vi "DSF.Engine.BuilderManager.Get Builder FIFO.vi"(11 "Builder Manager in":refnum<class "DSF.Engine.BuilderManager.lvclass">) -> (2 "Builder FIFO":refnum<k33>, 3 "Builder Manager out":refnum<class "DSF.Engine.BuilderManager.lvclass">)   [LabVIEW 2017, in "DSF.Engine.lvlib" / "DSF.Engine.BuilderManager.lvclass"]
uses:
  DSF.Engine.BuilderManager.lvclass
  DSF.Engine.BuilderManager.lvclass/DSF.Engine.BuilderManager.ctl
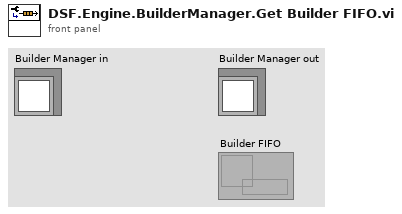
[diagram p1: front panel]
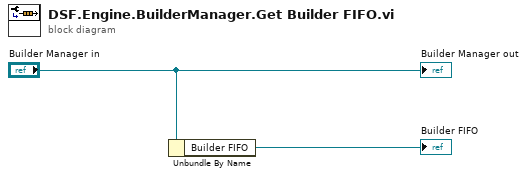
[diagram p0: block diagram]
diagram:
  n1 = Unbundle By Name("Builder Manager in") -> ("Builder FIFO"=→"Builder FIFO":refnum<k33>)
  "Builder Manager out" <- "Builder Manager in"
